vi "Get Engine Stream Filter.vi"(8 "error in (no error)":errorcluster, 11 "Refs":T4 {"Port Settings"."FD ISO Mode" items=["ISO", "Non ISO", "ISO Legacy"]; "Port Settings"."Termination" items=["Off", "On"]; "Port Settings"."Mode" items=["CAN 2.0", "CAN FD", "CAN FD+BRS"]}) -> (0 "error out":errorcluster, 3 "Filter":T3)   [LabVIEW 2019, in "CAN Stream Support Engine.lvlib"]
uses:
  CAN Stream Support Engine.lvlib
  Types/Engine Stream Refs.ctl
  Addon Shared/Types/Direction Filter.ctl
  Addon Shared/Types/Type Filter.ctl
  Addon Shared/Types/Filter Parameters.ctl
  Addon Shared/CAN Stream Support Shared.lvlib
  Types/Engine Stream Port Settings.ctl
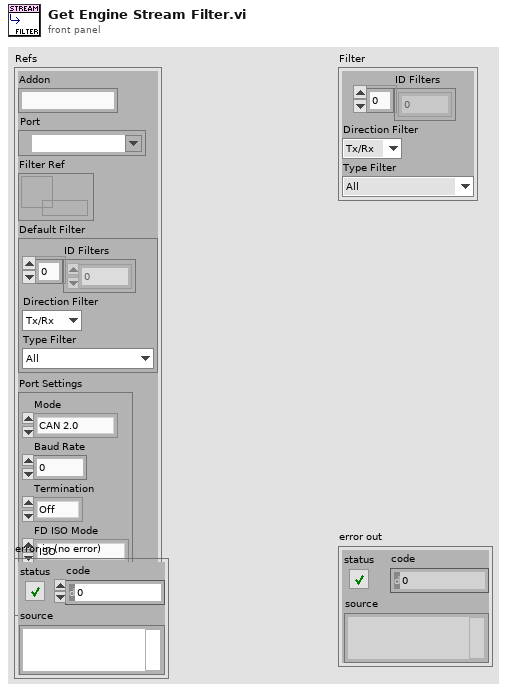
[diagram p1: front panel]
types:
  T1 = typedef "CAN Stream Support Shared.lvlib/Direction Filter.ctl" = enum16{"Tx/Rx", "Rx", "Tx"}
  T2 = typedef "CAN Stream Support Shared.lvlib/Type Filter.ctl" = enum16{"All", "CAN Data", "CAN Remote", "CAN Bus Error", "CAN 2.0 Data", "CAN FD Data", "CAN FD+BRS Data", "J1939 Data", "Delay", "Log Trigger", "Start Trigger"}
  T3 = cluster{"ID Filters":u32[], "Direction Filter":T1, "Type Filter":T2}
  T4 = typedef "CAN Stream Support Engine.lvlib/Engine Stream Refs.ctl" = cluster{"Addon":string, "Port":refnum<k21>, "Filter Ref":refnum<data-value>, "Default Filter":T5, "Port Settings":T6}
  T5 = typedef "CAN Stream Support Shared.lvlib/Filter Parameters.ctl" = cluster{"ID Filters":u32[], "Direction Filter":T1, "Type Filter":T2}
  T6 = typedef "Engine Stream Port Settings.ctl" = cluster{"Mode":u32, "Baud Rate":u64, "Termination":u32, "FD ISO Mode":u32, "FD Baud Rate":u64}
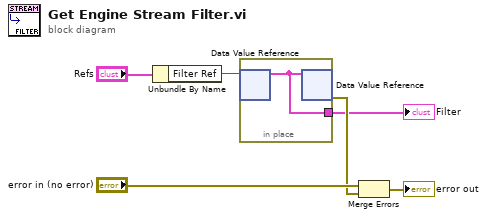
[diagram p0: block diagram]
diagram:
  n1 = Unbundle By Name("Refs") -> ("Filter Ref"=w5:refnum<data-value>)
  n2 = in-place {
    in-place-border: [w7] -> w1
    n3 = in-place-dvr #1(w5) -> (w7:T3)  [unwired: 1 out]
    n4 = in-place-dvr #1(w7) -> (w2:errorcluster)  [unwired: 1 out]
  }
  "Filter" <- w1
  n5 = Merge Errors("error in (no error)", w2) -> (→"error out":errorcluster)
